vi "Encoder_Lowpass_Filter.vi"(7 "LINK2_ENC_POS":dbl, 9 "LINK1_ENC_POS":dbl) -> (2 "LINK2_ENC_POS_FILTERED":dbl, 3 "LINK1_ENC_POS_FILTERED":dbl)   [LabVIEW 2017, in "myPAM.lvlib"]
uses:
  myPAM.lvlib
  <vilib>/Analysis/3filter.llb/Filter Passband Type.ctl
  <vilib>/Analysis/NI_AALBase.lvlib
  <vilib>/ptbypt/NI_PtbyPt.lvlib
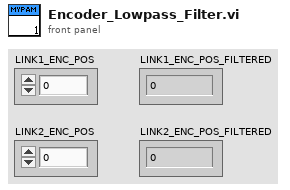
[diagram p1: front panel]
types:
  T1 = typedef "NI_AALBase.lvlib/Filter Passband Type.ctl" = enum32{"Lowpass", "Highpass", "Bandpass", "Bandstop"}
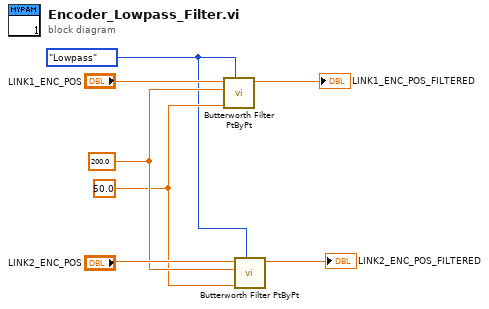
[diagram p0: block diagram]
diagram:
  w3 = Filter_Passband_Type."Lowpass" ("filter type")
  w4 = 50.0 ("low cutoff freq: fl")
  w5 = 200.0 ("sampling freq: fs")
  n1 = call <vilib>:"Butterworth Filter PtByPt.vi"("filter type"=w3, "low cutoff freq: fl"=w4, "sampling freq: fs"=w5, "x"="LINK1_ENC_POS") -> ("Filtered x"=→"LINK1_ENC_POS_FILTERED":dbl)  [unwired: 5 in, 1 out]
  n2 = call <vilib>:"Butterworth Filter PtByPt.vi"("filter type"=w3, "low cutoff freq: fl"=w4, "sampling freq: fs"=w5, "x"="LINK2_ENC_POS") -> ("Filtered x"=→"LINK2_ENC_POS_FILTERED":dbl)  [unwired: 5 in, 1 out]
